vi "Send Message and Wait for Response.vi"(4 "Timeout":i32, 6 "DataSocket Reply URL":string, 7 "Message Priority (Normal)":T1=enum."Normal", 8 "error in":errorcluster, 9 "Input":variant, 10 "Original Message":refnum<class "Reply Msg DataSocket Simple.lvclass">, 11 "Message Enqueuer in":refnum<class "Message Enqueuer.lvclass">) -> (0 "error out":errorcluster, 1 "Timeout?":bool, 2 "Reply":variant, 3 "Message Enqueuer out":refnum<class "Message Enqueuer.lvclass">)   [LabVIEW 2023, in "Reply Msg DataSocket Simple.lvclass"]
uses:
  Reply Msg DataSocket Simple.lvclass
  Reply Msg DataSocket Simple.lvclass/Reply Msg DataSocket Simple.ctl
  <vilib>/ActorFramework/Message Enqueuer/Message Enqueuer.lvclass
  <vilib>/ActorFramework/Message Enqueuer/Message Priority.ctl
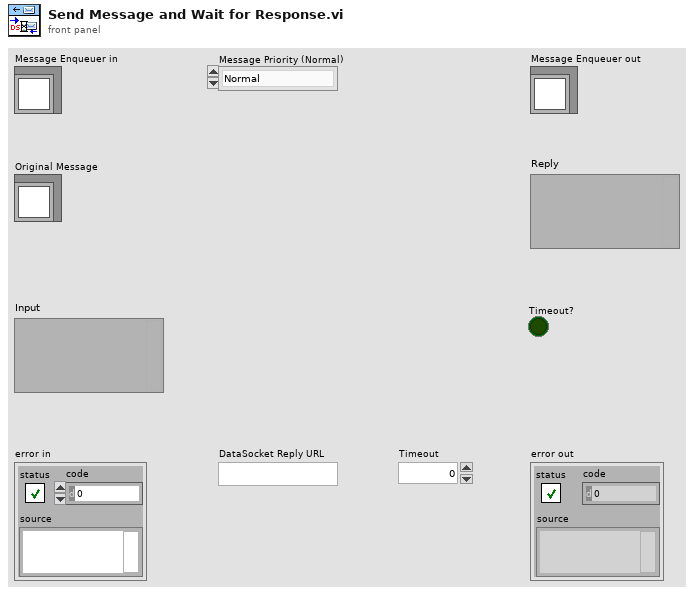
[diagram p1: front panel]
types:
  T1 = typedef "Actor Framework.lvlib/Message Enqueuer.lvclass/Message Priority.ctl" = enum16{"Low", "Normal", "High"}
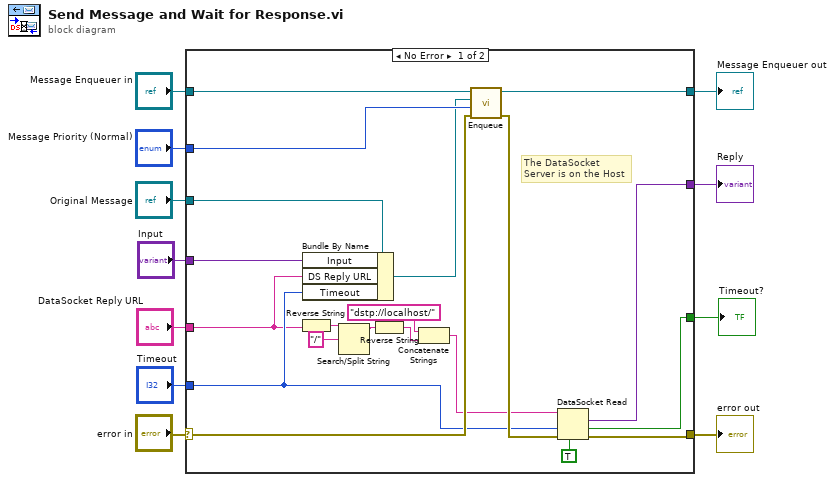
[diagram p0: block diagram]
diagram:
  n1 = case shown="No Error" "error in" {
    selector: "error in" -> [w28 w33]
    tunnel: [w24 w33] -> w6
    tunnel: "Original Message" -> [w27 _]
    tunnel: "Message Enqueuer in" -> [w31 w32]
    tunnel: [w22 _] -> w9
    tunnel: "Message Priority (Normal)" -> [w30 _]
    tunnel: [w29 w32] -> w8
    tunnel: [w23 _] -> w4
    tunnel: "Timeout" -> [w20 _]
    tunnel: "DataSocket Reply URL" -> [w18 _]
    tunnel: "Input" -> [w19 _]
    frame No Error {
      # "The DataSocket\nServer is on the Host"
      n2 = Reverse String(1:w18) -> (0:w17:string)
      n3 = Bundle By Name(cluster=w27, "Input"=w19, "DS Reply URL"=w18, "Timeout"=w20) -> (w26:refnum<class "Reply Msg DataSocket Simple.lvclass">)
      n4 = Search/Split String(string=w17, search string/char (-)="/") -> (substring before match=w12:string)  [unwired: 1 in, 2 out]
      n5 = Reverse String(1:w12) -> (0:w14:string)
      n6 = Concatenate Strings("dstp://localhost/" ("string"), w14) -> (w13:string)
      n7 = call <vilib>:"Enqueue.vi"("error in (no error)"=w28, "Message Priority (Normal)"=w30, "Message"=w26, "Message Enqueuer in"=w31) -> ("error out"=w25:errorcluster, "Message Enqueuer out"=w29:refnum<class "Message Enqueuer.lvclass">)  [unwired: 6 in]
      n8 = DataSocket Read(6:TRUE ("wait for updated value (T)"), 8:w25, 9:w20, 11:w13) -> (0:w24:errorcluster, 1:w23:bool, 2:w22:variant)  [unwired: 1 in, 4 out]
    }
    frame Error {
    }
  }
  "error out" <- w6
  "Reply" <- w9
  "Message Enqueuer out" <- w8
  "Timeout?" <- w4
